vi "EGEI.vi"() -> ()   [LabVIEW 2018]
uses:
  S4GEI/S4GEI.lvclass
  S4GEI/S4GEI.lvclass/S4GEI.ctl
  Request/Request.lvclass/Request.ctl
  Command/Command.lvclass/Command.ctl
  Channel GUI/Channel.lvclass
  Command/Command.lvclass
  Camera/Camera.lvclass
  Request/Request.lvclass
panel:
  in  "Tab Control 2":enum32{"Front Panel", "Setup Panel"}(tab)
  in  "Suffix":string
  in  "Start exposure":bool
  in  "Stop Acquisition":bool
  in  "Abort Acquisition":bool
  in  "Pause acquisition":bool
  in  "Exposure time":dbl=1.5 min=9.999999747378752e-06
  in  "Frames":u16=1 min=1 max=1000
  in  "Cycles":u32=1 min=1
  in  "PROPID":string="ENG"
  in  "Observer":string="Denis"
  in  "Object name":string="Test"
  in  "comment":string
  out "Cycles done":u16(slide)=1 max=2 scale=0.0..1.0
  out "Frames done":u16(slide)=1 max=2 scale=0.0..1.0
  out "CCD Status":string
  out "Exposing":bool
  out "Last image":string
  out "Temperature":i16
  out "Serial number":u16
  out "Current exp time":dbl
  out "Used disk":i16
  out "Power":bool
  out "ACS mode":bool
  in  "Device - Fiber set":u16(ring) items=["FIBER_SET"]
  in  "Action - Fiber set":u16(ring) items=["SET"]
  in  "Parameter - Fiber set":string
  in  "Send - Fiber set":bool
  in  "Device - Camera":u16(ring) items=["RED_CHANNEL", "BLUE_CHANNEL", "BOTH_CHANNELS"]
  in  "Action - Camera":u16(ring) items=["EXPOSE", "SET_EXPTIME", "SET_FRAMES", "SET_CYCLES", "SET_SUFFIX", "ABORT_ACQUISITION", "STOP_ACQUISITION", "STOP_APP"]
  in  "Parameter - Camera":string
  in  "Send - Camera":bool
  in  "OBJECT":bool caption="object"
  in  "TEST":bool caption="test"
  in  "ZERO":bool caption="zero"
  in  "DARK":bool caption="dark"
  in  "SFLAT":bool caption="sflat"
  in  "DFLAT":bool caption="dflat"
  in  "FOCUS":bool caption="focus"
  out "Error Message":string
  in  "Stop Application":bool
  in  "Channel ID":u16=1 min=1
  in  "ACS IP":string="200.131.64.25"
  in  "Final Line":u16=2048
  in  "Final Column":u16=2048
  in  "Initial Cloumn":u16=1
  in  "Initial Line":u16=1
  in  "Binning":u16=1
  in  "Shutter TTL":u16(ring) items=["TTL Low", "TTL High", "Error"]
  in  "Shutter Time":u16=50
  in  "Shutter Mode":u8(ring)=2 items=["OPEN"=1, "CLOSED"=2, "Error"=3]
  in  "AD Channel":u16
  in  "VShift Speed":u16(ring) items=["38.55", "76.95", "Error"]
  in  "Trigger Mode":u16(ring) items=["Internal", "External", "N/A", "N/A", "N/A", "N/A", "External Start", "External Exposure (Bulb)", "N/A", "External FVB EM", "Software", "N/A", "External Charge Shifting"]
  in  "Read Mode":u16(ring)=4 items=["Full Vertical Binning", "Multi-Track", "Random-Track", "Single-Track", "Image"]
  in  "Clock Amplitude":u16(ring) items=["Normal", "+1", "+2", "+3", "+4", "Error"]
  in  "Set camera configuration":bool
  in  "Temp":i32=20 min=-80 max=20
  in  "Cooler":bool
  in  "Sub Image":T1(radio)=enum."2048 x 2048"
  in  "High capacity":u16(ring) items=["Disabled", "Enabled"]
  in  "Readout Rate":u8(ring) items=["50 KHz", "1 MHz", "3 MHz", "5 MHz"]
  in  "Pre-amp gain":u8(ring) items=["Gain 1", "Gain 2", "Gain 4", "Error"]
  in  "Acquisition Mode":u16(ring)=3 items=["Reserved", "Single Scan", "Accumulate", "Kinetic", "Fast Kinetic", "Run till abort", "Reserved", "Reserved", "Reserved", "Time Delayed Integration"]
  # "ECHARPE Graphical Engineering Interface (EGEI)"
  # "Observation info"
  # "Request"
  # "Acquisition control"
  # "Pre-sets"
  # "Camera status"
  # "Errors"
  # "Camera operation mode"
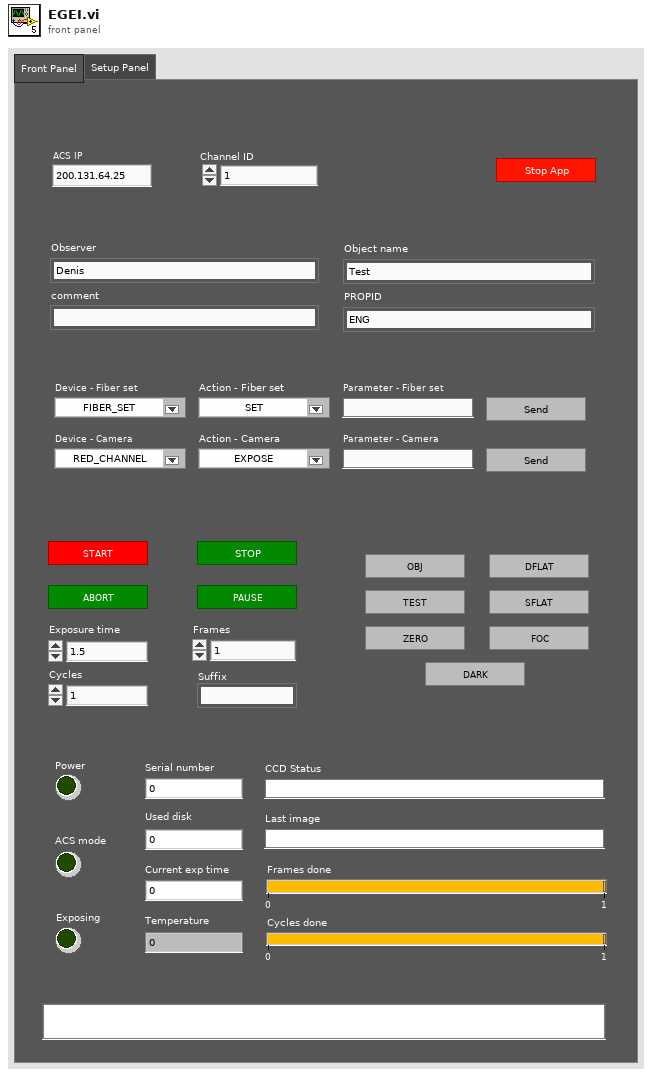
[diagram p1: front panel]
types:
  T1 = enum32{"512 x 512", "1024 x 1024", "Custom", "2048 x 2048"}
  T2 = cluster{"FWCS IP":string, "ACS IP":string, "Channel ID":u16}
  T3 = enum8{"Enabled", "Disabled", "Disabled and Grayed Out"}
  T4 = cluster{"CYCLES_DONE":u16, "LAST_IMAGE_NAME":string, "USED_DISK_SPACE":u16, "FRAMES_DONE":u16, "CCD_STATUS":string, "CURRENT_TEMPERATURE":i16, "TEMPERATURE_STATUS":string, "FRAME_EXPOSURE_TIME":sgl, "SERIAL_NUMBER":u16, "ACQUIRING":bool, "IMAGE_INDEX":u32, "POWER":bool, "ACS MODE":bool}
  T5 = cluster{"State Machine.lvclass":refnum<class "State Machine.lvclass">, "Channel.lvclass":refnum<class "Channel.lvclass">, "STATUS.lvclass":refnum<class "RxTx.lvclass">, "Status SM.lvclass":refnum<class "State Machine.lvclass">, "S4ICS.lvclass":refnum<class "S4ICS.lvclass">, "Acq State Machine.lvclass":refnum<class "State Machine.lvclass">, "Request SM.lvclass":refnum<class "State Machine.lvclass">, "Request.lvclass":refnum<class "Request.lvclass">}
  T6 = cluster{"device":string, "action":string, "parameter":string}
  T7 = cluster{"PREAMP":u16, "READOUT_RATE":u16, "VERTICAL_SHIFT_SPEED":u16, "READ_MODE":u16, "VERTICAL_CLOCK_VOLTAGE":u16, "ACQUISITION_MODE":u16, "AD_CHANNEL":u16, "SHUTTER_TTL":u16, "SHUTTER_OPENING_TIME":u16, "SHUTTER_CLOSING_TIME":u16, "SHUTTER_MODE":u16, "TRIGGER_MODE":u16, "VBIN":u16, "INITIAL_LINE":u16, "INITIAL_COLUMN":u16, "FINAL_LINE":u16, "FINAL_COLUMN":u16, "HBIN":u16, "HIGH_CAPACITY":bool, "COOLER":u16, "TEMP":u16}
  T8 = cluster{"EXPTIME":dbl, "#FRAMES":u32, "#CYCLES":u32, "suffix":string}
  T9 = cluster{"OBJECT":string, "OBSERVER":string, "CTRLINTE":string, "PROJID":string, "SYNCMODE":string, "INSTMODE":string, "FILTER":string, "OBSTYPE":string, "GUIVRSN":string, "COMMENT":string, "broker":string, "timestamp":string, "CHANNEL 1":bool, "CHANNEL 2":bool, "CHANNEL 3":bool, "CHANNEL 4":bool, "TCSMODE":bool}
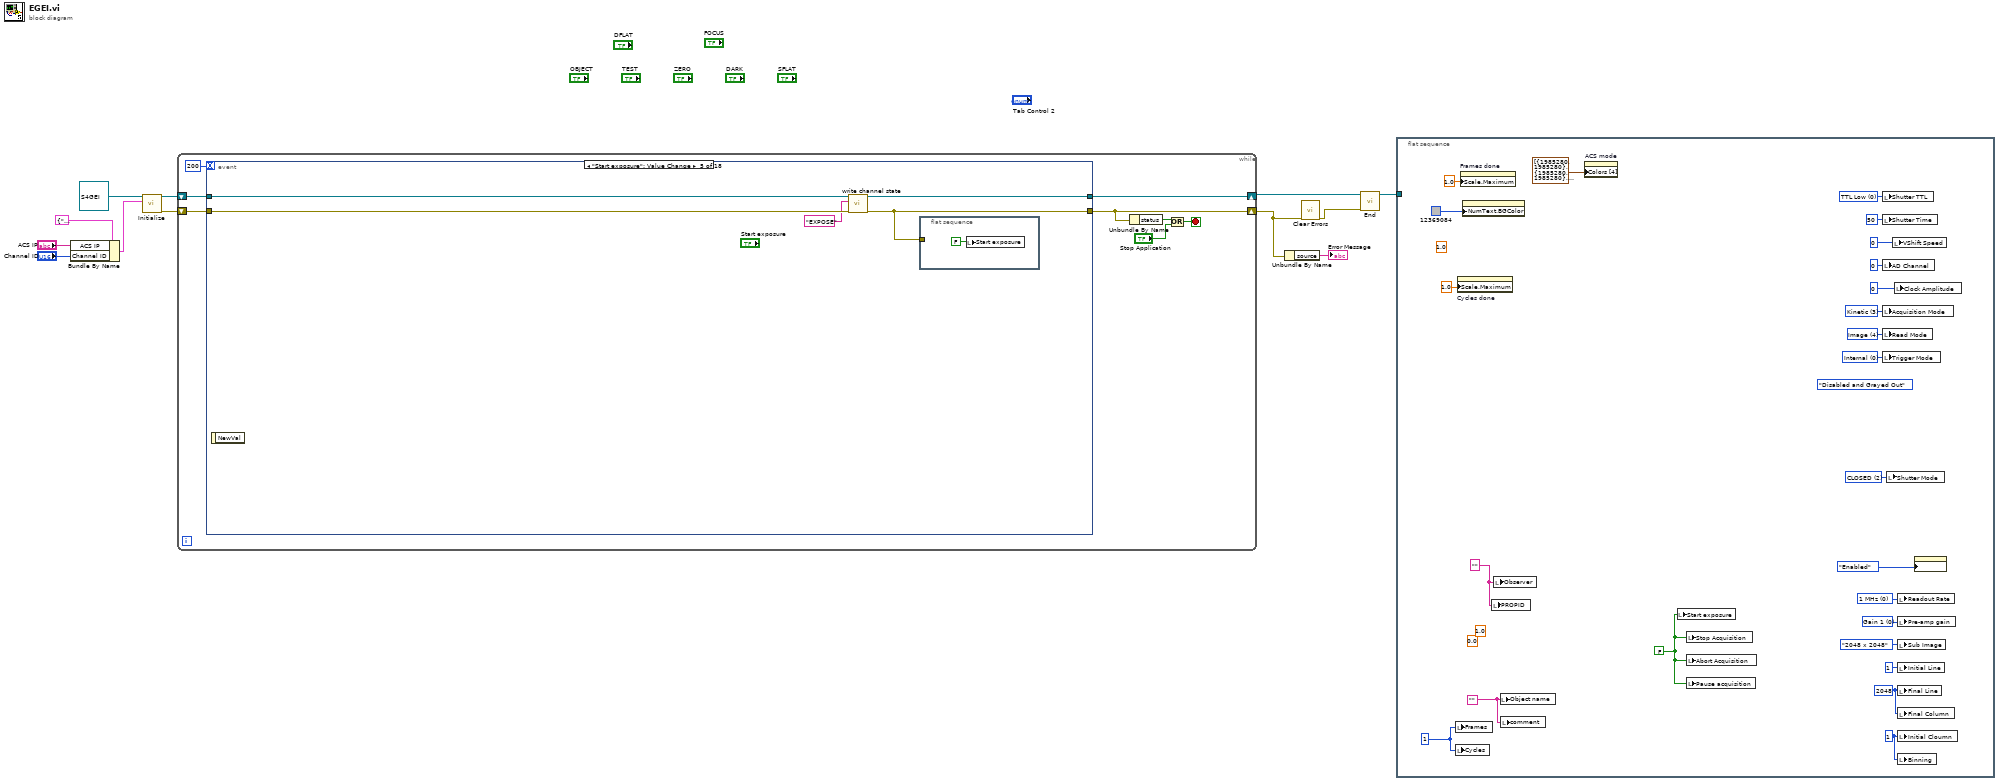
[diagram p0: block diagram]
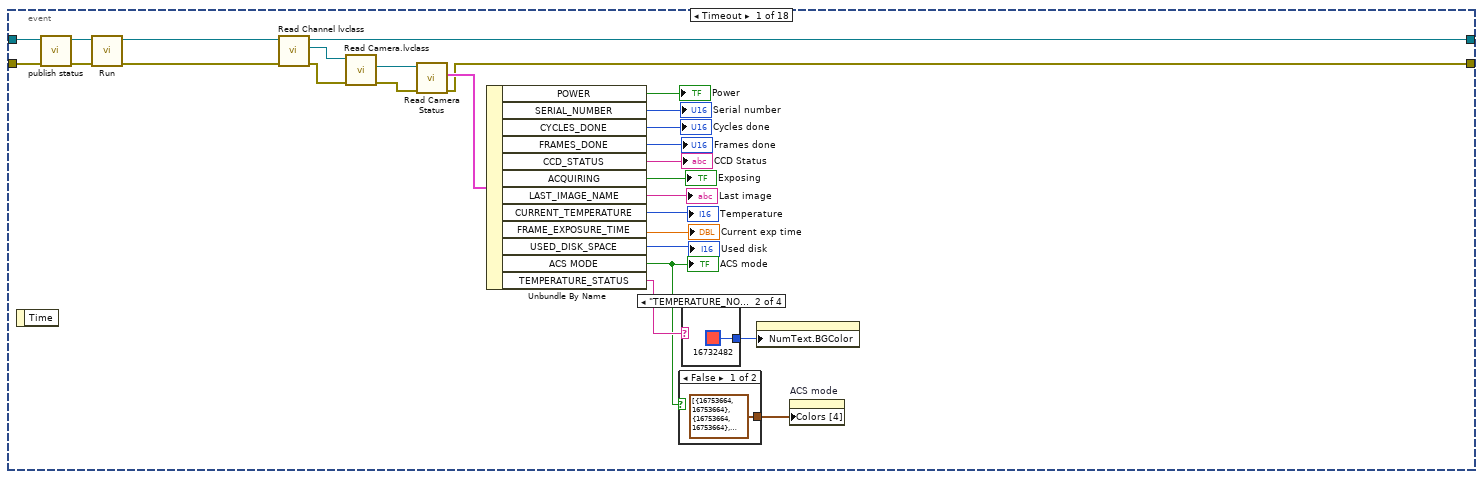
[diagram p2: hidden frame]
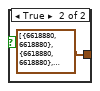
[diagram p3: hidden frame]
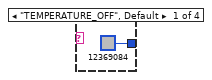
[diagram p4: hidden frame]
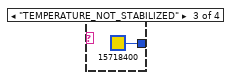
[diagram p5: hidden frame]
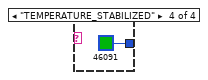
[diagram p6: hidden frame]
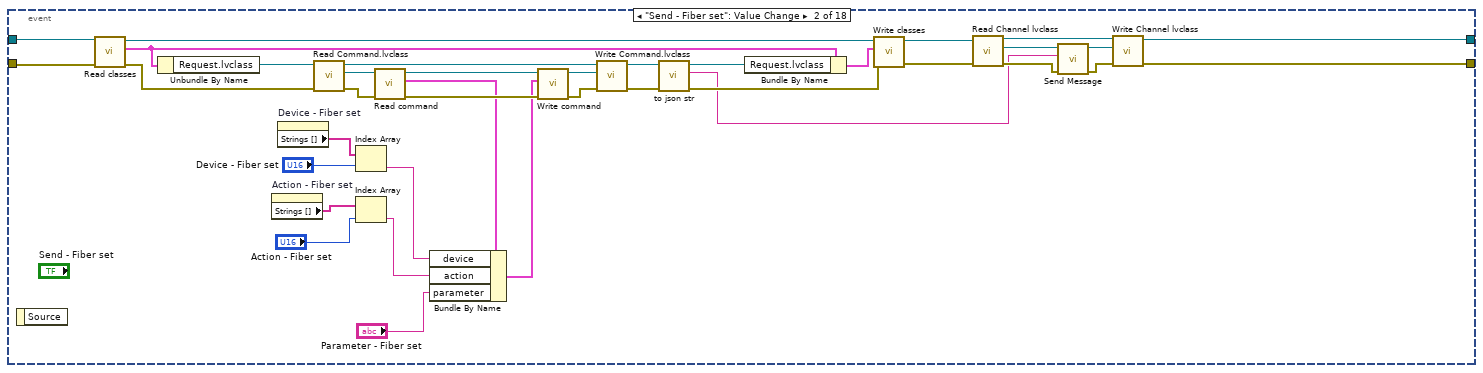
[diagram p7: hidden frame]
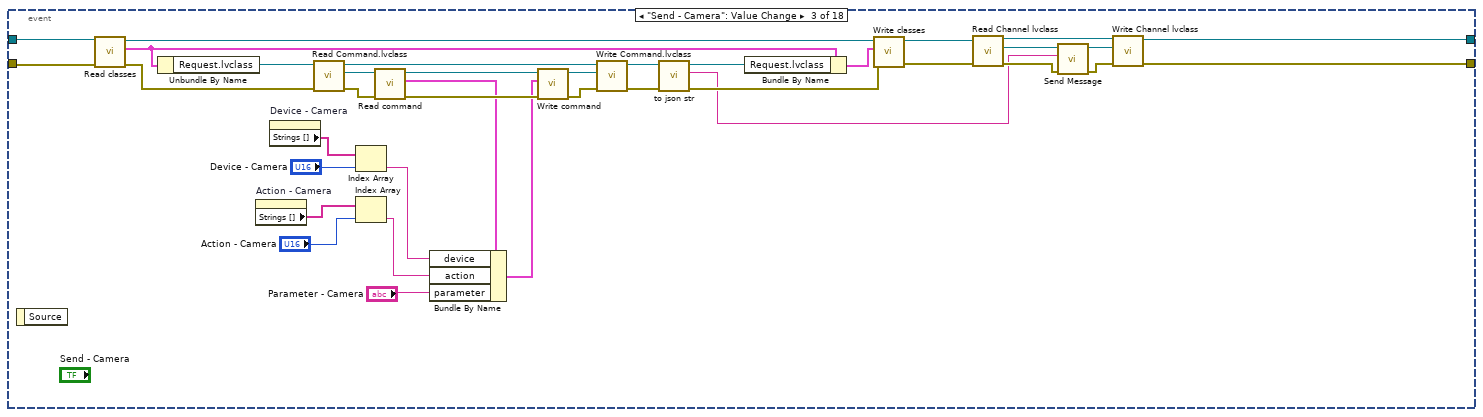
[diagram p8: hidden frame]
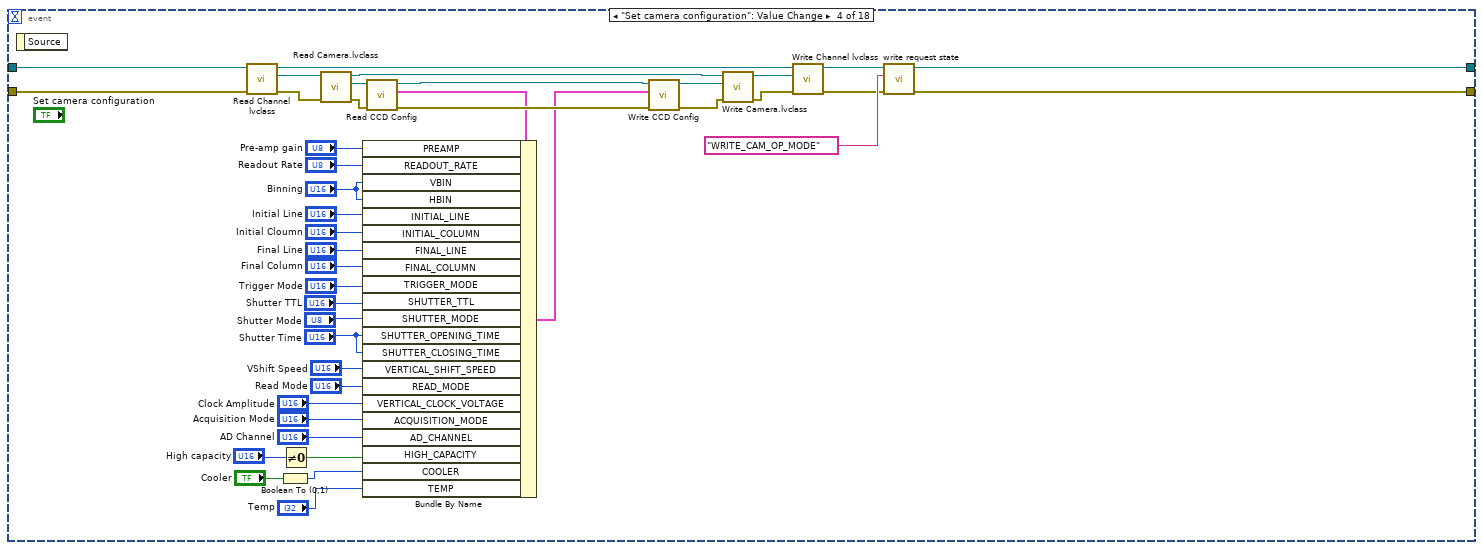
[diagram p9: hidden frame]
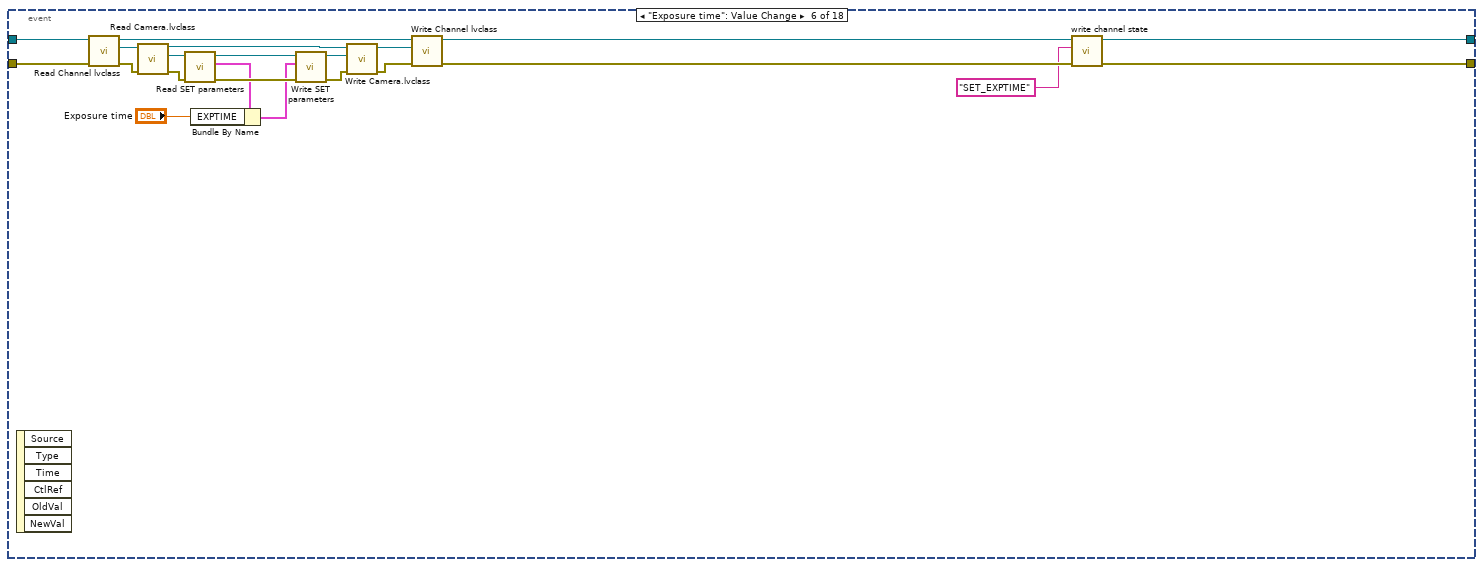
[diagram p10: hidden frame]
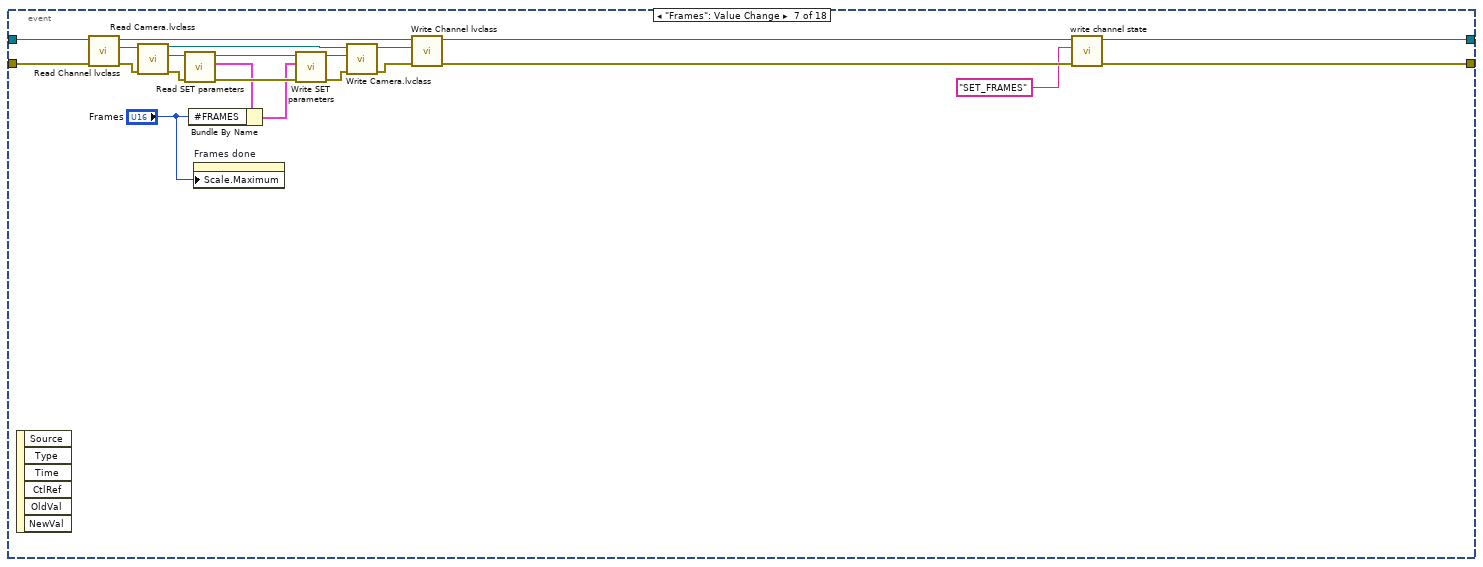
[diagram p11: hidden frame]
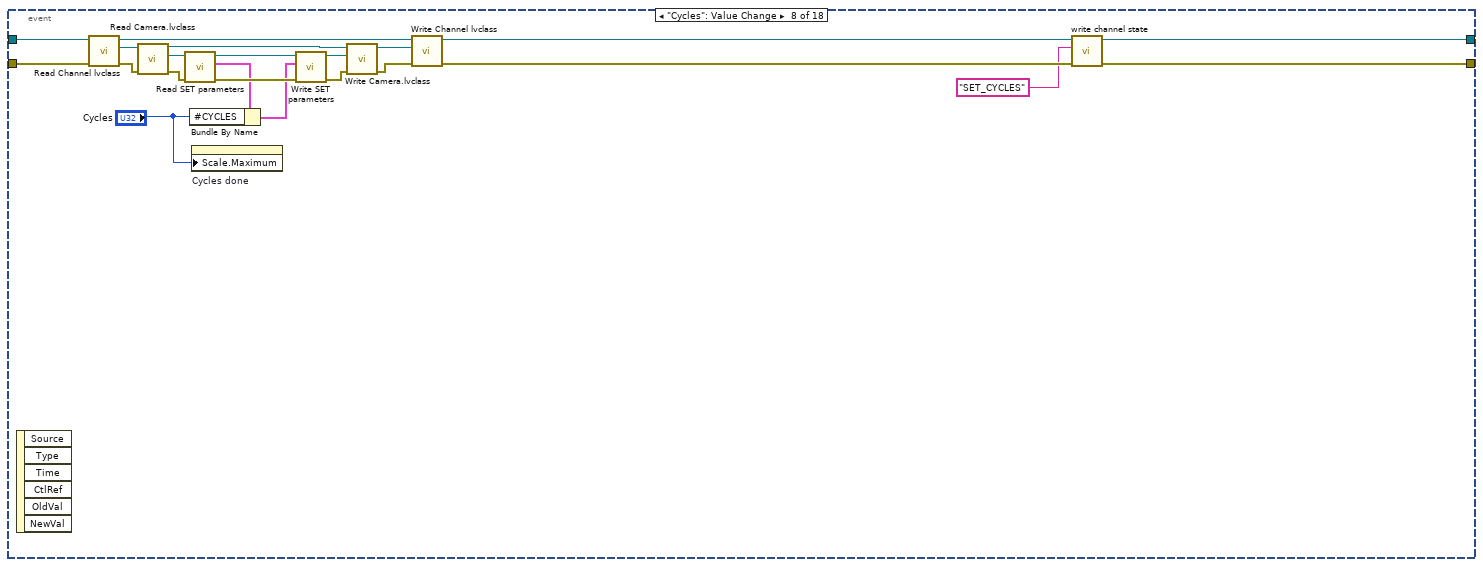
[diagram p12: hidden frame]
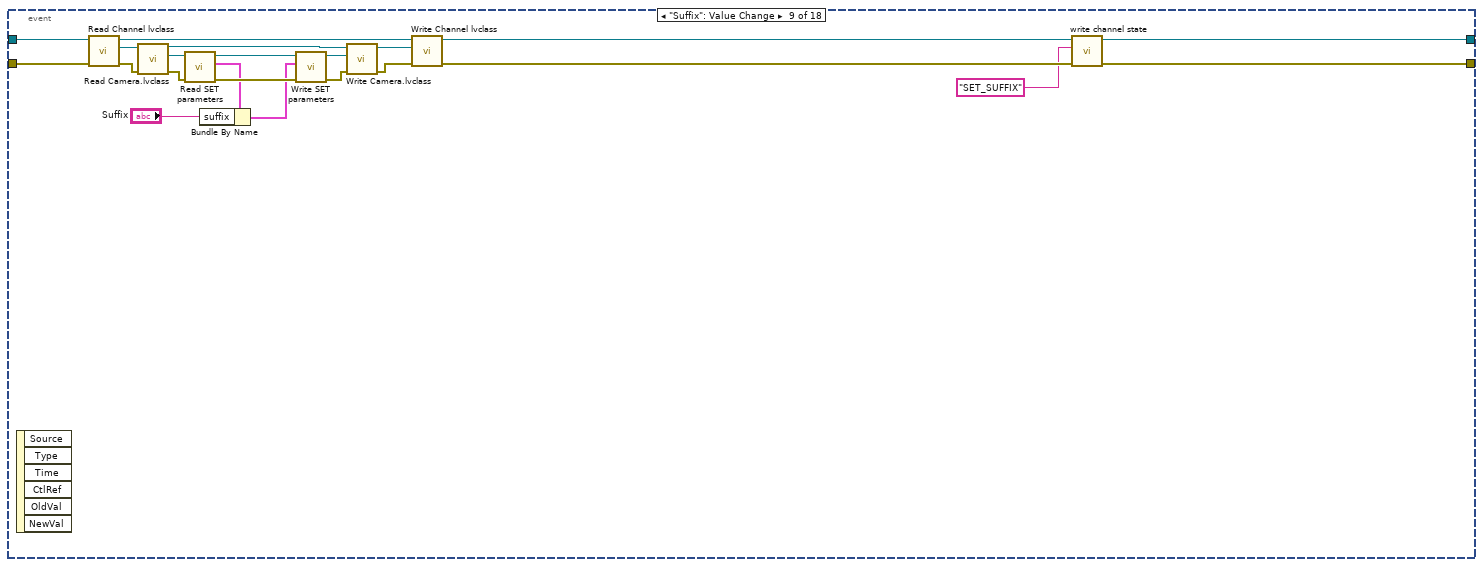
[diagram p13: hidden frame]
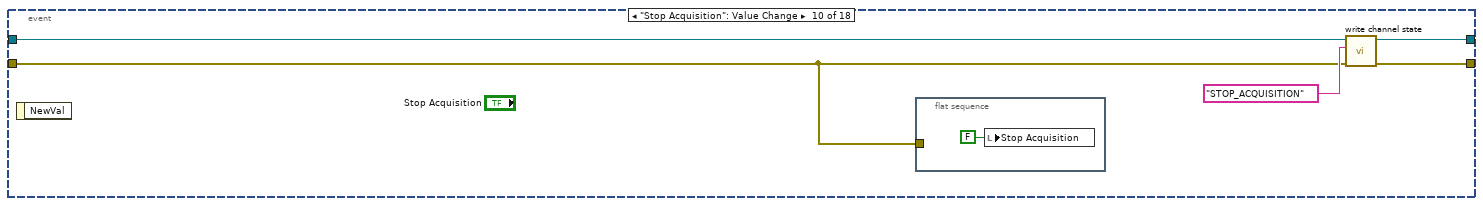
[diagram p14: hidden frame]
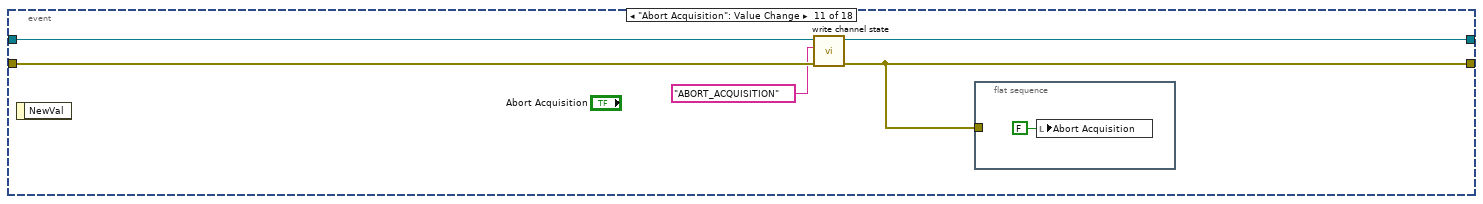
[diagram p15: hidden frame]
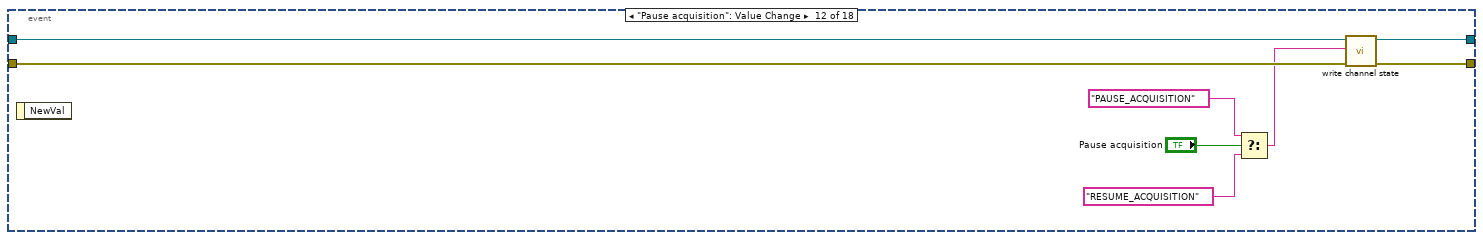
[diagram p16: hidden frame]
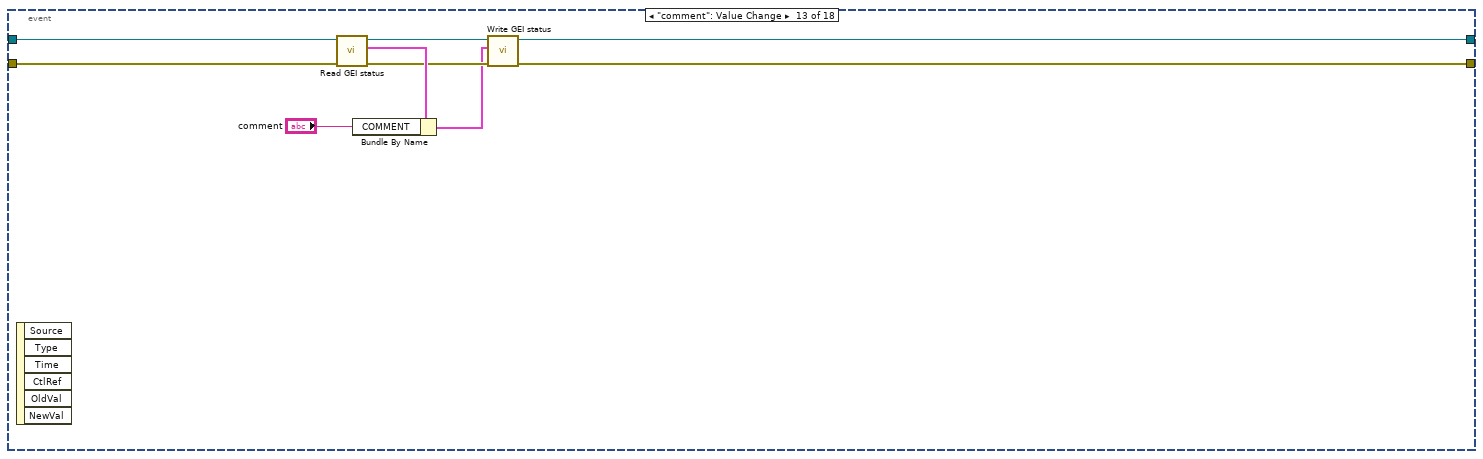
[diagram p17: hidden frame]
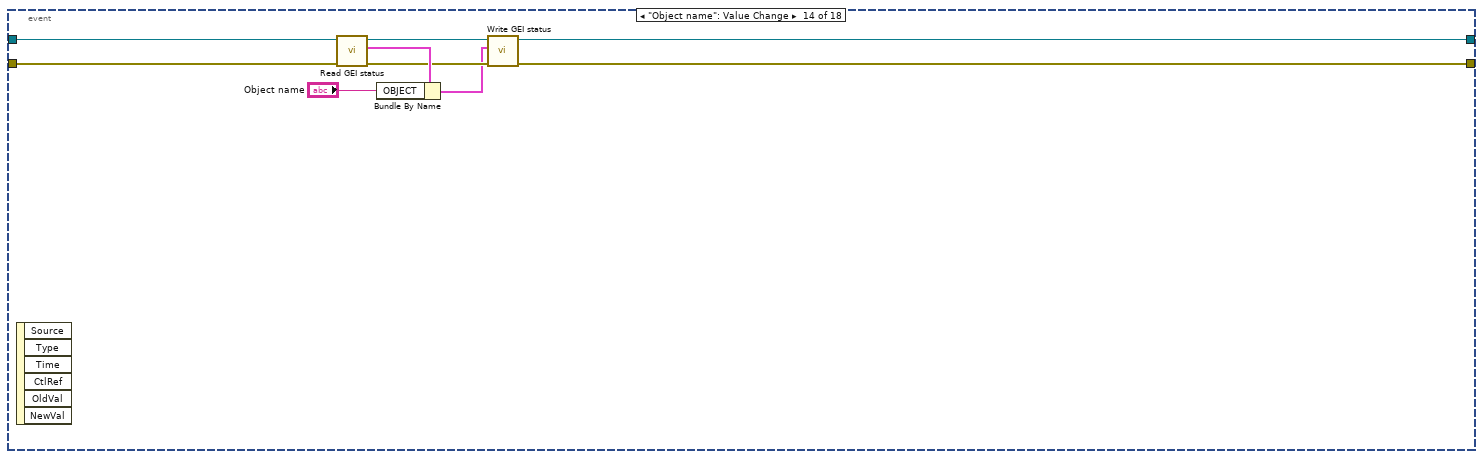
[diagram p18: hidden frame]
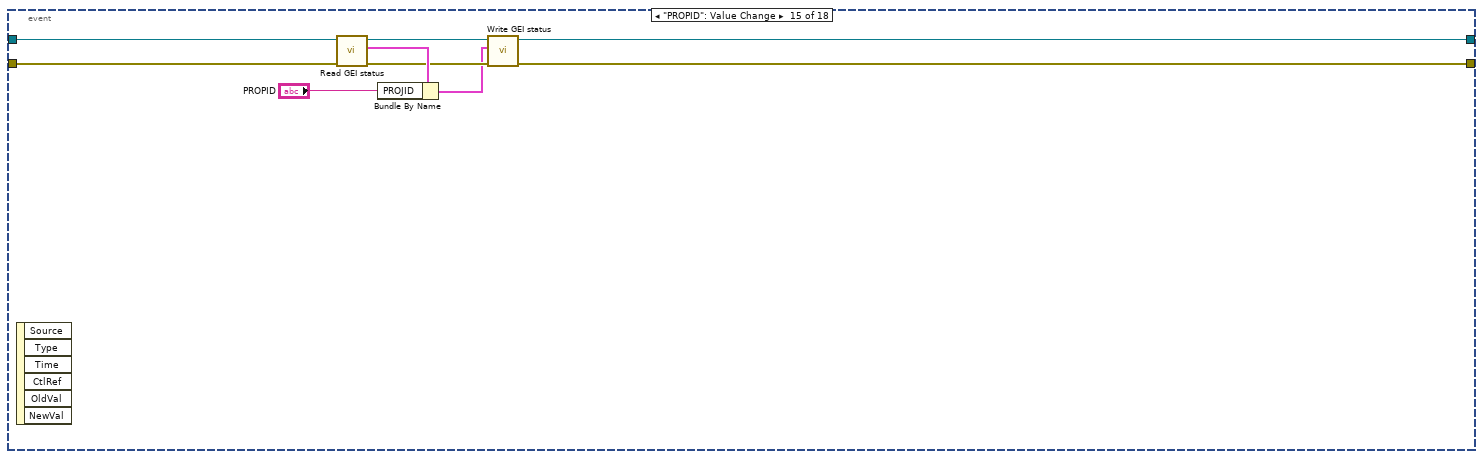
[diagram p19: hidden frame]
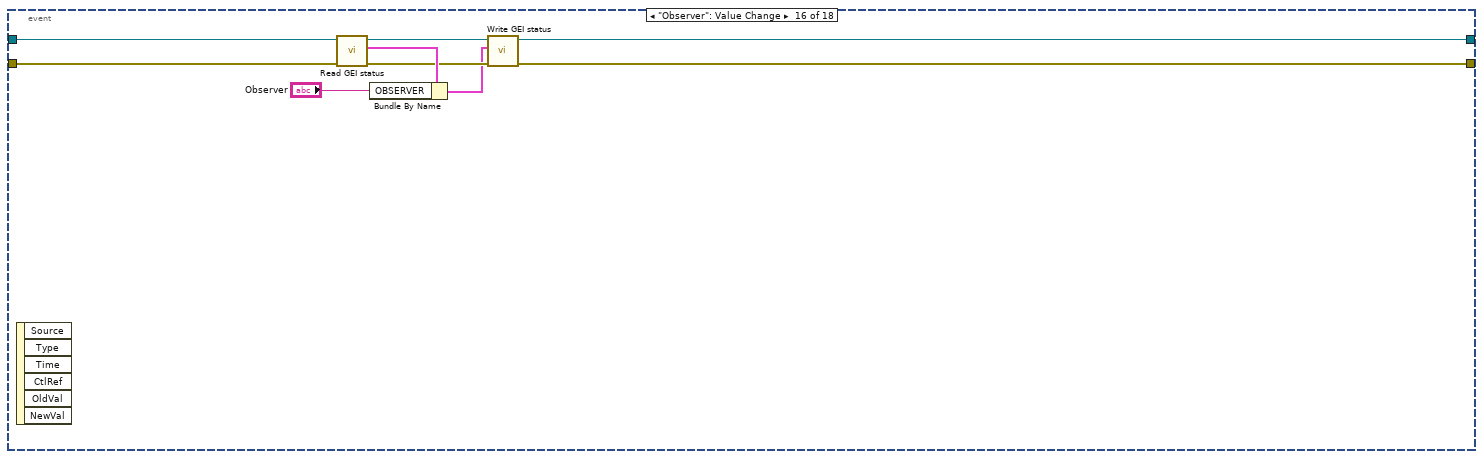
[diagram p20: hidden frame]
diagram:
  n1 = Bundle By Name(cluster=T2 {"FWCS IP"="200.131.64.49", "ACS IP"="200.131.64.25", "Channel ID"=1} ("Communication variables"), "ACS IP"="ACS IP", "Channel ID"="Channel ID") -> (w6:T2)
  n2 = call "Initialize.vi"("Communication variables"=w6, "SPARC4_GUI in"=refnum<class "S4GEI.lvclass"> refnum ("SPARC4_GUI.lvclass")) -> ("error out"=w2:errorcluster, "SPARC4_GUI out"=w1:refnum<class "S4GEI.lvclass">)  [unwired: 8 in]
  n3 = while {
    shift-right: [w13] -> w9
    shift-left: w2 -> [w15]
    shift-right: [w14] -> w11
    shift-left: w1 -> [w16]
    stop <- w19 stop-if-true
    n4 = event shown="[4] \"Start exposure\": Value Change" {
      selector: _ -> [_ _ _ _ _ _ _ _ _ _ _ _ _ _ _ _ _ _]
      dyn-events: _ -> [_ _ _ _ _ _ _ _ _ _ _ _ _ _ _ _ _ _]
      timeout: 200 -> [_ _ _ _ _ _ _ _ _ _ _ _ _ _ _ _ _ _]
      tunnel: w15 -> [w44 w70 w107 w168 w173 w195 w217 w239 w261 w264 w273 w282 w289 w298 w307 w316 w334 w357]
      tunnel: [w36 w84 w121 w134 w170 w177 w199 w221 w243 w266 w270 w280 w290 w299 w308 w317 w332 w357] -> w13
      tunnel: w16 -> [w45 w71 w108 w169 w174 w196 w218 w240 w262 w268 w274 w283 w291 w300 w309 w318 w335 w356]
      tunnel: [w37 w85 w122 w133 w171 w178 w200 w222 w244 w267 w272 w281 w292 w301 w310 w319 w333 w356] -> w14
      event Timeout {
        n5 = event-data() -> ()  [unwired: 1 in, 1 out]
        n6 = call "publish status.vi"("error in (no error)"=w44, "S4GEI in"=w45) -> ("error out"=w43:errorcluster, "S4GEI out"=w42:refnum<class "S4GEI.lvclass">)  [unwired: 8 in]
        n7 = call "Run.vi"("error in (no error)"=w43, "SPARC4_GUI in"=w42) -> ("error out"=w34:errorcluster, "SPARC4_GUI out"=w35:refnum<class "S4GEI.lvclass">)  [unwired: 8 in]
        n8 = call "Read Channel lvclass.vi"("error in (no error)"=w34, "SPARC4_GUI in"=w35) -> ("error out"=w39:errorcluster, "Channel.lvclass"=w41:refnum<class "Channel.lvclass">, "SPARC4_GUI out"=w37:refnum<class "S4GEI.lvclass">)  [unwired: 7 in]
        n9 = call-dynamic "Read Camera.lvclass.vi"("error in (no error)"=w39, "Channel in"=w41) -> ("error out"=w38:errorcluster, "Camera.lvclass"=w40:refnum<class "Camera.lvclass">)  [unwired: 7 in, 1 out]
        n10 = call-dynamic "Read Camera Status.vi"("error in (no error)"=w38, "Camera in"=w40) -> ("error out"=w36:errorcluster, "camera status"=w46:T4)  [unwired: 7 in, 1 out]
        n11 = Unbundle By Name(w46) -> ("POWER"=→"Power":bool, "SERIAL_NUMBER"=→"Serial number":u16, "CYCLES_DONE"=→"Cycles done":u16, "FRAMES_DONE"=→"Frames done":u16, "CCD_STATUS"=→"CCD Status":string, "ACQUIRING"=→"Exposing":bool, "LAST_IMAGE_NAME"=→"Last image":string, "CURRENT_TEMPERATURE"=→"Temperature":i16, "FRAME_EXPOSURE_TIME"=→"Current exp time":sgl, "USED_DISK_SPACE"=→"Used disk":u16, "ACS MODE"=w29:bool, "TEMPERATURE_STATUS"=w33:string)
        "ACS mode" <- w29
        n12 = case shown="False" w29 {
          tunnel: [cluster{u32, u32}[] [{16753664, 16753664}, {16753664, 16753664}, {16753664, 16753664}] ("Colors [4]") cluster{u32, u32}[] [{6618880, 6618880}, {6618880, 6618880}, {6618880, 6618880}] ("Colors [4]")] -> w32
          frame False {
          }
          frame True {
          }
        }
        n13 = case shown="\"TEMPERATURE_NOT_REACHED\"" w33 {
          tunnel: [u32 12369084 u32 16732482 u32 15718400 u32 46091] -> w47
          frame "TEMPERATURE_OFF", Default {
          }
          frame "TEMPERATURE_NOT_REACHED" {
          }
          frame "TEMPERATURE_NOT_STABILIZED" {
          }
          frame "TEMPERATURE_STABILIZED" {
          }
        }
        n14 = property on="Temperature" class="DigNum (strict)"("NumText.BGColor"=w47) -> ()  [unwired: 2 in, 2 out]
        n15 = property on="ACS mode" class="Bool (strict)"("Colors [4]"=w32) -> ()  [unwired: 2 in, 2 out]
      }
      event "Send - Fiber set": Value Change {
        n16 = event-data() -> ()  [unwired: 1 in, 1 out]
        n17 = call-dynamic "Read classes.vi"("error in (no error)"=w70, "S4GEI in"=w71) -> ("error out"=w72:errorcluster, "classes"=w81:T5, "S4GEI out"=w79:refnum<class "S4GEI.lvclass">)  [unwired: 7 in]
        n18 = Unbundle By Name(w81) -> ("Request.lvclass"=w83:refnum<class "Request.lvclass">)
        n19 = property on="Action - Fiber set" class="Ring (strict)"() -> ("Strings []"=w56:string[])  [unwired: 2 in, 2 out]
        n20 = property on="Device - Fiber set" class="Ring (strict)"() -> ("Strings []"=w59:string[])  [unwired: 2 in, 2 out]
        n21 = call "Read Command.lvclass.vi"("error in (no error)"=w72, "Request in"=w83) -> ("error out"=w73:errorcluster, "Command.lvclass"=w78:refnum<class "Command.lvclass">, "Request out"=w82:refnum<class "Request.lvclass">)  [unwired: 7 in]
        n22 = Index Array(array=w59, index="Device - Fiber set") -> (element=w58:string)
        n23 = Index Array(array=w56, index="Action - Fiber set") -> (element=w54:string)
        n24 = call "Read command.vi"("error in (no error)"=w73, "Command in"=w78) -> ("error out"=w74:errorcluster, "command"=w67:T6, "Command out"=w77:refnum<class "Command.lvclass">)  [unwired: 7 in]
        n25 = Bundle By Name(cluster=w67, "device"=w58, "action"=w54, "parameter"="Parameter - Fiber set") -> (w66:T6)
        n26 = call "Write command.vi"("error in (no error)"=w74, "command"=w66, "Command in"=w77) -> ("error out"=w75:errorcluster, "Command out"=w76:refnum<class "Command.lvclass">)  [unwired: 7 in]
        n27 = call "Write Command.lvclass.vi"("error in (no error)"=w75, "Command.lvclass"=w76, "Request in"=w82) -> ("error out"=w63:errorcluster, "Request out"=w64:refnum<class "Request.lvclass">)  [unwired: 7 in]
        n28 = call "to json str.vi"("error in (no error)"=w63, "Request in"=w64) -> ("error out"=w62:errorcluster, "request str"=w60:string, "Request out"=w61:refnum<class "Request.lvclass">)  [unwired: 7 in]
        n29 = Bundle By Name(cluster=w81, "Request.lvclass"=w61) -> (w80:T5)
        n30 = call-dynamic "Write classes.vi"("error in (no error)"=w62, "classes"=w80, "S4GEI in"=w79) -> ("error out"=w68:errorcluster, "S4GEI out"=w69:refnum<class "S4GEI.lvclass">)  [unwired: 7 in]
        n31 = call "Read Channel lvclass.vi"("error in (no error)"=w68, "SPARC4_GUI in"=w69) -> ("error out"=w87:errorcluster, "Channel.lvclass"=w90:refnum<class "Channel.lvclass">, "SPARC4_GUI out"=w86:refnum<class "S4GEI.lvclass">)  [unwired: 7 in]
        n32 = call "Send Message.vi"("error in (no error)"=w87, "Message"=w60, "Channel GUI in"=w90) -> ("error out"=w88:errorcluster, "Channel GUI out"=w89:refnum<class "Channel.lvclass">)  [unwired: 7 in]
        n33 = call "Write Channel lvclass.vi"("error in (no error)"=w88, "Channel.lvclass"=w89, "SPARC4_GUI in"=w86) -> ("error out"=w84:errorcluster, "SPARC4_GUI out"=w85:refnum<class "S4GEI.lvclass">)  [unwired: 7 in]
      }
      event "Send - Camera": Value Change {
        n34 = event-data() -> ()  [unwired: 1 in, 1 out]
        n35 = call-dynamic "Read classes.vi"("error in (no error)"=w107, "S4GEI in"=w108) -> ("error out"=w109:errorcluster, "classes"=w118:T5, "S4GEI out"=w116:refnum<class "S4GEI.lvclass">)  [unwired: 7 in]
        n36 = Unbundle By Name(w118) -> ("Request.lvclass"=w120:refnum<class "Request.lvclass">)
        n37 = property on="Action - Camera" class="Ring (strict)"() -> ("Strings []"=w93:string[])  [unwired: 2 in, 2 out]
        n38 = property on="Device - Camera" class="Ring (strict)"() -> ("Strings []"=w95:string[])  [unwired: 2 in, 2 out]
        n39 = call "Read Command.lvclass.vi"("error in (no error)"=w109, "Request in"=w120) -> ("error out"=w110:errorcluster, "Command.lvclass"=w115:refnum<class "Command.lvclass">, "Request out"=w119:refnum<class "Request.lvclass">)  [unwired: 7 in]
        n40 = Index Array(array=w95, index="Device - Camera") -> (element=w91:string)
        n41 = Index Array(array=w93, index="Action - Camera") -> (element=w92:string)
        n42 = call "Read command.vi"("error in (no error)"=w110, "Command in"=w115) -> ("error out"=w111:errorcluster, "command"=w104:T6, "Command out"=w114:refnum<class "Command.lvclass">)  [unwired: 7 in]
        n43 = Bundle By Name(cluster=w104, "device"=w91, "action"=w92, "parameter"="Parameter - Camera") -> (w103:T6)
        n44 = call "Write command.vi"("error in (no error)"=w111, "command"=w103, "Command in"=w114) -> ("error out"=w112:errorcluster, "Command out"=w113:refnum<class "Command.lvclass">)  [unwired: 7 in]
        n45 = call "Write Command.lvclass.vi"("error in (no error)"=w112, "Command.lvclass"=w113, "Request in"=w119) -> ("error out"=w101:errorcluster, "Request out"=w102:refnum<class "Request.lvclass">)  [unwired: 7 in]
        n46 = call "to json str.vi"("error in (no error)"=w101, "Request in"=w102) -> ("error out"=w100:errorcluster, "request str"=w98:string, "Request out"=w99:refnum<class "Request.lvclass">)  [unwired: 7 in]
        n47 = Bundle By Name(cluster=w118, "Request.lvclass"=w99) -> (w117:T5)
        n48 = call-dynamic "Write classes.vi"("error in (no error)"=w100, "classes"=w117, "S4GEI in"=w116) -> ("error out"=w105:errorcluster, "S4GEI out"=w106:refnum<class "S4GEI.lvclass">)  [unwired: 7 in]
        n49 = call "Read Channel lvclass.vi"("error in (no error)"=w105, "SPARC4_GUI in"=w106) -> ("error out"=w124:errorcluster, "Channel.lvclass"=w127:refnum<class "Channel.lvclass">, "SPARC4_GUI out"=w123:refnum<class "S4GEI.lvclass">)  [unwired: 7 in]
        n50 = call "Send Message.vi"("error in (no error)"=w124, "Message"=w98, "Channel GUI in"=w127) -> ("error out"=w125:errorcluster, "Channel GUI out"=w126:refnum<class "Channel.lvclass">)  [unwired: 7 in]
        n51 = call "Write Channel lvclass.vi"("error in (no error)"=w125, "Channel.lvclass"=w126, "SPARC4_GUI in"=w123) -> ("error out"=w121:errorcluster, "SPARC4_GUI out"=w122:refnum<class "S4GEI.lvclass">)  [unwired: 7 in]
      }
      event "Set camera configuration": Value Change {
        n52 = event-data() -> ()  [unwired: 1 in, 1 out]
        n53 = call "Read Channel lvclass.vi"("error in (no error)"=w168, "SPARC4_GUI in"=w169) -> ("error out"=w167:errorcluster, "Channel.lvclass"=w139:refnum<class "Channel.lvclass">, "SPARC4_GUI out"=w166:refnum<class "S4GEI.lvclass">)  [unwired: 7 in]
        n54 = Boolean To (0,1)(Boolean="Cooler") -> (0, 1=w131:i16)
        n55 = Not Equal To 0?(x="High capacity") -> (x != 0?=w128:bool)
        n56 = call-dynamic "Read Camera.lvclass.vi"("error in (no error)"=w167, "Channel in"=w139) -> ("error out"=w165:errorcluster, "Camera.lvclass"=w164:refnum<class "Camera.lvclass">, "Channel out"=w138:refnum<class "Channel.lvclass">)  [unwired: 7 in]
        n57 = call-dynamic "Read CCD Config.vi"("error in (no error)"=w165, "Camera in"=w164) -> ("error out"=w163:errorcluster, "CCD Config"=w141:T7, "Camera out"=w146:refnum<class "Camera.lvclass">)  [unwired: 7 in]
        n58 = Bundle By Name(cluster=w141, "PREAMP"="Pre-amp gain", "READOUT_RATE"="Readout Rate", "VBIN"="Binning", "HBIN"="Binning", "INITIAL_LINE"="Initial Line", "INITIAL_COLUMN"="Initial Cloumn", "FINAL_LINE"="Final Line", "FINAL_COLUMN"="Final Column", "TRIGGER_MODE"="Trigger Mode", "SHUTTER_TTL"="Shutter TTL", "SHUTTER_MODE"="Shutter Mode", "SHUTTER_OPENING_TIME"="Shutter Time", "SHUTTER_CLOSING_TIME"="Shutter Time", "VERTICAL_SHIFT_SPEED"="VShift Speed", "READ_MODE"="Read Mode", "VERTICAL_CLOCK_VOLTAGE"="Clock Amplitude", "ACQUISITION_MODE"="Acquisition Mode", "AD_CHANNEL"="AD Channel", "HIGH_CAPACITY"=w128, "COOLER"=w131, "TEMP"="Temp") -> (w140:T7)
        n59 = call-dynamic "Write CCD Config.vi"("error in (no error)"=w163, "CCD Config"=w140, "Camera in"=w146) -> ("error out"=w144:errorcluster, "Camera out"=w145:refnum<class "Camera.lvclass">)  [unwired: 7 in]
        n60 = call-dynamic "Write Camera.lvclass.vi"("error in (no error)"=w144, "Camera.lvclass"=w145, "Channel in"=w138) -> ("error out"=w143:errorcluster, "Channel out"=w142:refnum<class "Channel.lvclass">)  [unwired: 7 in]
        n61 = call "Write Channel lvclass.vi"("error in (no error)"=w143, "Channel.lvclass"=w142, "SPARC4_GUI in"=w166) -> ("error out"=w136:errorcluster, "SPARC4_GUI out"=w135:refnum<class "S4GEI.lvclass">)  [unwired: 7 in]
        n62 = call "write request state.vi"("error in (no error)"=w136, "State"="WRITE_CAM_OP_MODE", "S4GEI in"=w135) -> ("error out"=w134:errorcluster, "S4GEI out"=w133:refnum<class "S4GEI.lvclass">)  [unwired: 7 in]
      }
      event "Start exposure": Value Change {
        n63 = event-data() -> ()  [unwired: 1 in, 1 out]
        n64 = call "write channel state.vi"("error in (no error)"=w173, "State"="EXPOSE", "S4GEI in"=w174) -> ("error out"=w170:errorcluster, "S4GEI out"=w171:refnum<class "S4GEI.lvclass">)  [unwired: 7 in]
        n65 = flat-sequence {
          tunnel: w170 -> [_]
          frame #0 {
            n66 = local write "Start exposure"(FALSE ("Start exposure")) -> ()
          }
        }
      }
      event "Exposure time": Value Change {
        n67 = event-data() -> ()  [unwired: 1 in, 6 out]
        n68 = call "Read Channel lvclass.vi"("error in (no error)"=w195, "SPARC4_GUI in"=w196) -> ("error out"=w194:errorcluster, "Channel.lvclass"=w183:refnum<class "Channel.lvclass">, "SPARC4_GUI out"=w197:refnum<class "S4GEI.lvclass">)  [unwired: 7 in]
        n69 = call-dynamic "Read Camera.lvclass.vi"("error in (no error)"=w194, "Channel in"=w183) -> ("error out"=w190:errorcluster, "Camera.lvclass"=w191:refnum<class "Camera.lvclass">, "Channel out"=w182:refnum<class "Channel.lvclass">)  [unwired: 7 in]
        n70 = call-dynamic "Read SET parameters.vi"("error in (no error)"=w190, "Camera in"=w191) -> ("error out"=w188:errorcluster, "SET parameters"=w185:T8, "Camera out"=w189:refnum<class "Camera.lvclass">)  [unwired: 7 in]
        n71 = Bundle By Name(cluster=w185, "EXPTIME"="Exposure time") -> (w184:T8)
        n72 = call-dynamic "Write SET parameters.vi"("error in (no error)"=w188, "SET parameters"=w184, "Camera in"=w189) -> ("error out"=w186:errorcluster, "Camera out"=w187:refnum<class "Camera.lvclass">)  [unwired: 7 in]
        n73 = call-dynamic "Write Camera.lvclass.vi"("error in (no error)"=w186, "Camera.lvclass"=w187, "Channel in"=w182) -> ("error out"=w193:errorcluster, "Channel out"=w192:refnum<class "Channel.lvclass">)  [unwired: 7 in]
        n74 = call "Write Channel lvclass.vi"("error in (no error)"=w193, "Channel.lvclass"=w192, "SPARC4_GUI in"=w197) -> ("error out"=w180:errorcluster, "SPARC4_GUI out"=w181:refnum<class "S4GEI.lvclass">)  [unwired: 7 in]
        n75 = call "write channel state.vi"("error in (no error)"=w180, "State"="SET_EXPTIME", "S4GEI in"=w181) -> ("error out"=w177:errorcluster, "S4GEI out"=w178:refnum<class "S4GEI.lvclass">)  [unwired: 7 in]
      }
      event "Frames": Value Change {
        n76 = event-data() -> ()  [unwired: 1 in, 6 out]
        n77 = call "Read Channel lvclass.vi"("error in (no error)"=w217, "SPARC4_GUI in"=w218) -> ("error out"=w216:errorcluster, "Channel.lvclass"=w205:refnum<class "Channel.lvclass">, "SPARC4_GUI out"=w219:refnum<class "S4GEI.lvclass">)  [unwired: 7 in]
        n78 = call-dynamic "Read Camera.lvclass.vi"("error in (no error)"=w216, "Channel in"=w205) -> ("error out"=w212:errorcluster, "Camera.lvclass"=w213:refnum<class "Camera.lvclass">, "Channel out"=w204:refnum<class "Channel.lvclass">)  [unwired: 7 in]
        n79 = call-dynamic "Read SET parameters.vi"("error in (no error)"=w212, "Camera in"=w213) -> ("error out"=w210:errorcluster, "SET parameters"=w207:T8, "Camera out"=w211:refnum<class "Camera.lvclass">)  [unwired: 7 in]
        n80 = Bundle By Name(cluster=w207, "#FRAMES"="Frames") -> (w206:T8)
        n81 = property on="Frames done" class="Slide (strict)"("Scale.Maximum"="Frames") -> ()  [unwired: 2 in, 2 out]
        n82 = call-dynamic "Write SET parameters.vi"("error in (no error)"=w210, "SET parameters"=w206, "Camera in"=w211) -> ("error out"=w208:errorcluster, "Camera out"=w209:refnum<class "Camera.lvclass">)  [unwired: 7 in]
        n83 = call-dynamic "Write Camera.lvclass.vi"("error in (no error)"=w208, "Camera.lvclass"=w209, "Channel in"=w204) -> ("error out"=w215:errorcluster, "Channel out"=w214:refnum<class "Channel.lvclass">)  [unwired: 7 in]
        n84 = call "Write Channel lvclass.vi"("error in (no error)"=w215, "Channel.lvclass"=w214, "SPARC4_GUI in"=w219) -> ("error out"=w202:errorcluster, "SPARC4_GUI out"=w203:refnum<class "S4GEI.lvclass">)  [unwired: 7 in]
        n85 = call "write channel state.vi"("error in (no error)"=w202, "State"="SET_FRAMES", "S4GEI in"=w203) -> ("error out"=w199:errorcluster, "S4GEI out"=w200:refnum<class "S4GEI.lvclass">)  [unwired: 7 in]
      }
      event "Cycles": Value Change {
        n86 = event-data() -> ()  [unwired: 1 in, 6 out]
        n87 = call "Read Channel lvclass.vi"("error in (no error)"=w239, "SPARC4_GUI in"=w240) -> ("error out"=w238:errorcluster, "Channel.lvclass"=w227:refnum<class "Channel.lvclass">, "SPARC4_GUI out"=w241:refnum<class "S4GEI.lvclass">)  [unwired: 7 in]
        n88 = call-dynamic "Read Camera.lvclass.vi"("error in (no error)"=w238, "Channel in"=w227) -> ("error out"=w234:errorcluster, "Camera.lvclass"=w235:refnum<class "Camera.lvclass">, "Channel out"=w226:refnum<class "Channel.lvclass">)  [unwired: 7 in]
        n89 = call-dynamic "Read SET parameters.vi"("error in (no error)"=w234, "Camera in"=w235) -> ("error out"=w232:errorcluster, "SET parameters"=w229:T8, "Camera out"=w233:refnum<class "Camera.lvclass">)  [unwired: 7 in]
        n90 = Bundle By Name(cluster=w229, "#CYCLES"="Cycles") -> (w228:T8)
        n91 = property on="Cycles done" class="Slide (strict)"("Scale.Maximum"="Cycles") -> ()  [unwired: 2 in, 2 out]
        n92 = call-dynamic "Write SET parameters.vi"("error in (no error)"=w232, "SET parameters"=w228, "Camera in"=w233) -> ("error out"=w230:errorcluster, "Camera out"=w231:refnum<class "Camera.lvclass">)  [unwired: 7 in]
        n93 = call-dynamic "Write Camera.lvclass.vi"("error in (no error)"=w230, "Camera.lvclass"=w231, "Channel in"=w226) -> ("error out"=w237:errorcluster, "Channel out"=w236:refnum<class "Channel.lvclass">)  [unwired: 7 in]
        n94 = call "Write Channel lvclass.vi"("error in (no error)"=w237, "Channel.lvclass"=w236, "SPARC4_GUI in"=w241) -> ("error out"=w224:errorcluster, "SPARC4_GUI out"=w225:refnum<class "S4GEI.lvclass">)  [unwired: 7 in]
        n95 = call "write channel state.vi"("error in (no error)"=w224, "State"="SET_CYCLES", "S4GEI in"=w225) -> ("error out"=w221:errorcluster, "S4GEI out"=w222:refnum<class "S4GEI.lvclass">)  [unwired: 7 in]
      }
      event "Suffix": Value Change {
        n96 = event-data() -> ()  [unwired: 1 in, 6 out]
        n97 = call "Read Channel lvclass.vi"("error in (no error)"=w261, "SPARC4_GUI in"=w262) -> ("error out"=w260:errorcluster, "Channel.lvclass"=w249:refnum<class "Channel.lvclass">, "SPARC4_GUI out"=w263:refnum<class "S4GEI.lvclass">)  [unwired: 7 in]
        n98 = call-dynamic "Read Camera.lvclass.vi"("error in (no error)"=w260, "Channel in"=w249) -> ("error out"=w256:errorcluster, "Camera.lvclass"=w257:refnum<class "Camera.lvclass">, "Channel out"=w248:refnum<class "Channel.lvclass">)  [unwired: 7 in]
        n99 = call-dynamic "Read SET parameters.vi"("error in (no error)"=w256, "Camera in"=w257) -> ("error out"=w254:errorcluster, "SET parameters"=w251:T8, "Camera out"=w255:refnum<class "Camera.lvclass">)  [unwired: 7 in]
        n100 = Bundle By Name(cluster=w251, "suffix"="Suffix") -> (w250:T8)
        n101 = call-dynamic "Write SET parameters.vi"("error in (no error)"=w254, "SET parameters"=w250, "Camera in"=w255) -> ("error out"=w252:errorcluster, "Camera out"=w253:refnum<class "Camera.lvclass">)  [unwired: 7 in]
        n102 = call-dynamic "Write Camera.lvclass.vi"("error in (no error)"=w252, "Camera.lvclass"=w253, "Channel in"=w248) -> ("error out"=w259:errorcluster, "Channel out"=w258:refnum<class "Channel.lvclass">)  [unwired: 7 in]
        n103 = call "Write Channel lvclass.vi"("error in (no error)"=w259, "Channel.lvclass"=w258, "SPARC4_GUI in"=w263) -> ("error out"=w246:errorcluster, "SPARC4_GUI out"=w247:refnum<class "S4GEI.lvclass">)  [unwired: 7 in]
        n104 = call "write channel state.vi"("error in (no error)"=w246, "State"="SET_SUFFIX", "S4GEI in"=w247) -> ("error out"=w243:errorcluster, "S4GEI out"=w244:refnum<class "S4GEI.lvclass">)  [unwired: 7 in]
      }
      event "Stop Acquisition": Value Change {
        n105 = event-data() -> ()  [unwired: 1 in, 1 out]
        n106 = flat-sequence {
          tunnel: w264 -> [_]
          frame #0 {
            n107 = local write "Stop Acquisition"(FALSE ("Stop Acquisition")) -> ()
          }
        }
        n108 = call "write channel state.vi"("error in (no error)"=w264, "State"="STOP_ACQUISITION", "S4GEI in"=w268) -> ("error out"=w266:errorcluster, "S4GEI out"=w267:refnum<class "S4GEI.lvclass">)  [unwired: 7 in]
      }
      event "Abort Acquisition": Value Change {
        n109 = event-data() -> ()  [unwired: 1 in, 1 out]
        n110 = call "write channel state.vi"("error in (no error)"=w273, "State"="ABORT_ACQUISITION", "S4GEI in"=w274) -> ("error out"=w270:errorcluster, "S4GEI out"=w272:refnum<class "S4GEI.lvclass">)  [unwired: 7 in]
        n111 = flat-sequence {
          tunnel: w270 -> [_]
          frame #0 {
            n112 = local write "Abort Acquisition"(FALSE ("Abort Acquisition")) -> ()
          }
        }
      }
      event "Pause acquisition": Value Change {
        n113 = event-data() -> ()  [unwired: 1 in, 1 out]
        n114 = Select(t="PAUSE_ACQUISITION", s="Pause acquisition", f="RESUME_ACQUISITION") -> (s? t:f=w278:string)
        n115 = call "write channel state.vi"("error in (no error)"=w282, "State"=w278, "S4GEI in"=w283) -> ("error out"=w280:errorcluster, "S4GEI out"=w281:refnum<class "S4GEI.lvclass">)  [unwired: 7 in]
      }
      event "comment": Value Change {
        n116 = event-data() -> ()  [unwired: 1 in, 6 out]
        n117 = call-dynamic "Read GEI status.vi"("error in (no error)"=w289, "S4GEI in"=w291) -> ("error out"=w287:errorcluster, "GEI status"=w288:T9, "S4GEI out"=w286:refnum<class "S4GEI.lvclass">)  [unwired: 7 in]
        n118 = Bundle By Name(cluster=w288, "COMMENT"="comment") -> (w285:T9)
        n119 = call-dynamic "Write GEI status.vi"("error in (no error)"=w287, "GEI status"=w285, "S4GEI in"=w286) -> ("error out"=w290:errorcluster, "S4GEI out"=w292:refnum<class "S4GEI.lvclass">)  [unwired: 7 in]
      }
      event "Object name": Value Change {
        n120 = event-data() -> ()  [unwired: 1 in, 6 out]
        n121 = call-dynamic "Read GEI status.vi"("error in (no error)"=w298, "S4GEI in"=w300) -> ("error out"=w296:errorcluster, "GEI status"=w297:T9, "S4GEI out"=w295:refnum<class "S4GEI.lvclass">)  [unwired: 7 in]
        n122 = Bundle By Name(cluster=w297, "OBJECT"="Object name") -> (w294:T9)
        n123 = call-dynamic "Write GEI status.vi"("error in (no error)"=w296, "GEI status"=w294, "S4GEI in"=w295) -> ("error out"=w299:errorcluster, "S4GEI out"=w301:refnum<class "S4GEI.lvclass">)  [unwired: 7 in]
      }
      event "PROPID": Value Change {
        n124 = event-data() -> ()  [unwired: 1 in, 6 out]
        n125 = call-dynamic "Read GEI status.vi"("error in (no error)"=w307, "S4GEI in"=w309) -> ("error out"=w305:errorcluster, "GEI status"=w306:T9, "S4GEI out"=w304:refnum<class "S4GEI.lvclass">)  [unwired: 7 in]
        n126 = Bundle By Name(cluster=w306, "PROJID"="PROPID") -> (w303:T9)
        n127 = call-dynamic "Write GEI status.vi"("error in (no error)"=w305, "GEI status"=w303, "S4GEI in"=w304) -> ("error out"=w308:errorcluster, "S4GEI out"=w310:refnum<class "S4GEI.lvclass">)  [unwired: 7 in]
      }
      event "Observer": Value Change {
        n128 = event-data() -> ()  [unwired: 1 in, 6 out]
        n129 = call-dynamic "Read GEI status.vi"("error in (no error)"=w316, "S4GEI in"=w318) -> ("error out"=w314:errorcluster, "GEI status"=w315:T9, "S4GEI out"=w313:refnum<class "S4GEI.lvclass">)  [unwired: 7 in]
        n130 = Bundle By Name(cluster=w315, "OBSERVER"="Observer") -> (w312:T9)
        n131 = call-dynamic "Write GEI status.vi"("error in (no error)"=w314, "GEI status"=w312, "S4GEI in"=w313) -> ("error out"=w317:errorcluster, "S4GEI out"=w319:refnum<class "S4GEI.lvclass">)  [unwired: 7 in]
      }
      event "Sub Image": Value Change {
        n132 = event-data() -> ()  [unwired: 1 in, 1 out]
        n133 = Divide(x=2048, y=2) -> (x/y=w320:dbl)
        n134 = case shown="\"512 x 512\"" "Sub Image" {
          tunnel: [256 512 1024 512] -> w326
          frame "512 x 512" {
          }
          frame "1024 x 1024" {
          }
          frame "2048 x 2048", Default {
          }
          frame "Custom" {
          }
        }
        n135 = case shown="\"Custom\"" "Sub Image" {
          tunnel: [T3."Disabled and Grayed Out" ("Disabled") T3."Enabled" ("Disabled")] -> w329
          frame "1024 x 1024", Default {
          }
          frame "Custom" {
          }
        }
        n136 = Add(x=w320, y=w326) -> (x+y=w322:dbl)
        n137 = Subtract(x=w320, y=w326) -> (x-y=w327:dbl)
        n138 = Subtract(x=w320, y=w326) -> (x-y=w328:dbl)
        n139 = Add(x=w320, y=w326) -> (x+y=w331:dbl)
        n140 = Increment(x=w327) -> (x+1=w330:dbl)
        n141 = Increment(x=w328) -> (x+1=w323:dbl)
        n142 = local write "Initial Cloumn"(w330) -> ()
        n143 = local write "Final Column"(w331) -> ()
        n144 = local write "Initial Line"(w323) -> ()
        n145 = local write "Final Line"(w322) -> ()
        n146 = property on="Initial Line" class="DigNum (strict)"("DisabledEnum"=w329) -> ()  [unwired: 2 in, 2 out]
        n147 = property on="Initial Cloumn" class="DigNum (strict)"("DisabledEnum"=w329) -> ()  [unwired: 2 in, 2 out]
        n148 = property on="Final Line" class="DigNum (strict)"("DisabledEnum"=w329) -> ()  [unwired: 2 in, 2 out]
        n149 = property on="Final Column" class="DigNum (strict)"("DisabledEnum"=w329) -> ()  [unwired: 2 in, 2 out]
        n150 = flat-sequence {
          tunnel: w334 -> [w352]
          tunnel: w335 -> [w353]
          tunnel: [w353] -> w333
          tunnel: [w352] -> w332
          frame #0 {
            w346 = cluster{dbl, dbl} {0.0, 0.0}
            n151 = local read "Initial Cloumn"() -> (w345:u16)
            n152 = local read "Final Column"() -> (w343:u16)
            n153 = local read "Final Line"() -> (w344:u16)
            n154 = local read "Final Line"() -> (w342:u16)
            n155 = Bundle(cluster=w346, w345, w344) -> (w351:cluster{dbl, dbl})
            n156 = Bundle(cluster=w346, w345, w342) -> (w350:cluster{dbl, dbl})
            n157 = Bundle(cluster=w346, w343, w342) -> (w349:cluster{dbl, dbl})
            n158 = Bundle(cluster=w346, w343, w344) -> (w348:cluster{dbl, dbl})
            n159 = Bundle(cluster=w346, w345, w344) -> (w347:cluster{dbl, dbl})
            n160 = Build Array(w351, w350, w349, w348, w347) -> ()  [unwired: 1 out]
          }
        }
      }
      event "Acquisition Mode": Value Change {
        n161 = event-data() -> ("NewVal"=w355:u16)  [unwired: 1 in]
        n162 = case shown="1, Default" w355 {
          tunnel: [T3."Enabled" ("Disabled") T3."Disabled and Grayed Out" ("Disabled")] -> w354
          frame 3 {
          }
          frame 1, Default {
          }
        }
        n163 = property on="Frames" class="DigNum (strict)"("DisabledEnum"=w354) -> ()  [unwired: 2 in, 2 out]
      }
    }
    n164 = Unbundle By Name(w13) -> ("status"=w18:bool)
    n165 = Or(x=w18, y="Stop Application") -> (x .or. y?=w19:bool)
  }
  n166 = Unbundle By Name(w9) -> ("source"=→"Error Message":string)
  n167 = call <vilib>:"Clear Errors.vi"("error in (no error)"=w9) -> ("error out"=w8:errorcluster)  [unwired: 5 in, 1 out]
  n168 = call "End.vi"("error in (no error)"=w8, "SPARC4_GUI in"=w11) -> ("SPARC4_GUI out"=w12:refnum<class "S4GEI.lvclass">)  [unwired: 8 in, 1 out]
  n169 = flat-sequence {
    tunnel: w12 -> [_]
    frame #0 {
      w362 = 1
      w364 = ""
      w365 = FALSE ("analyser status")
      (unwired) 0.0 ("Scale.Range:Minimum")
      (unwired) 1.0 ("Scale.Range:Maximum")
      (unwired) 1.0 ("Scale.Range:Maximum")
      (unwired) T3."Disabled and Grayed Out" ("Disabled")
      w369 = u16 0 items=["Internal", "External", "N/A", "N/A", "N/A", "N/A", "External Start", "External Exposure (Bulb)", "N/A", "External FVB EM", "Software", "N/A", "External Charge Shifting"] ("Trigger Mode")
      w370 = u16 4 items=["Full Vertical Binning", "Multi-Track", "Random-Track", "Single-Track", "Image"] ("Read Mode")
      w371 = u16 3 items=["Reserved", "Single Scan", "Accumulate", "Kinetic", "Fast Kinetic", "Run till abort", "Reserved", "Reserved", "Reserved", "Time Delayed Integration"] ("Acquisition Mode")
      w376 = u16 0 items=["TTL Low", "TTL High"] ("Shutter TTL")
      w377 = u8 0 items=["  1 MHz", "0.1 MHz"] ("Readout Rate")
      w379 = u8 2 items=["Fully Auto", "OPEN", "CLOSED"] ("Shutter Mode")
      w363 = "" ("Command:")
      w381 = u16 2048 ("Final Line")
      w380 = u16 1 ("Initial Cloumn")
      w383 = u8 0 items=["Gain 1", "Gain 2"] ("Pre-amp gain")
      n170 = local write "Frames"(w362) -> ()
      n171 = local write "Cycles"(w362) -> ()
      n172 = property on="Cycles done" class="Slide (strict)"("Scale.Maximum"=1.0 ("Scale.Range:Maximum")) -> ()  [unwired: 2 in, 2 out]
      n173 = property on="Frames done" class="Slide (strict)"("Scale.Maximum"=1.0 ("Scale.Range:Maximum")) -> ()  [unwired: 2 in, 2 out]
      n174 = property on="Temperature" class="DigNum (strict)"("NumText.BGColor"=u32 12369084) -> ()  [unwired: 2 in, 2 out]
      n175 = local write "PROPID"(w363) -> ()
      n176 = local write "Observer"(w363) -> ()
      n177 = local write "Object name"(w364) -> ()
      n178 = local write "comment"(w364) -> ()
      n179 = property on="ACS mode" class="Bool (strict)"("Colors [4]"=cluster{u32, u32}[] [{1985280, 1985280}, {1985280, 1985280}, {6618880, 6618880}]) -> ()  [unwired: 2 in, 2 out]
      n180 = local write "Start exposure"(w365) -> ()
      n181 = local write "Stop Acquisition"(w365) -> ()
      n182 = local write "Abort Acquisition"(w365) -> ()
      n183 = local write "Pause acquisition"(w365) -> ()
      n184 = local write "Shutter TTL"(w376) -> ()
      n185 = local write "Shutter Time"(u16 50 ("Shutter Time")) -> ()
      n186 = local write "AD Channel"(u16 0 ("AD Channel")) -> ()
      n187 = local write "Acquisition Mode"(w371) -> ()
      n188 = local write "Read Mode"(w370) -> ()
      n189 = local write "Trigger Mode"(w369) -> ()
      n190 = local write "Shutter Mode"(w379) -> ()
      n191 = local write "VShift Speed"(u16 0 ("Vertical Shift Speed")) -> ()
      n192 = local write "Clock Amplitude"(u16 0 ("Vertical Clock Voltagem")) -> ()
      n193 = local write "Readout Rate"(w377) -> ()
      n194 = local write "Pre-amp gain"(w383) -> ()
      n195 = local write "Sub Image"(T1."2048 x 2048" ("Sub Image")) -> ()
      n196 = local write "Initial Line"(u16 1 ("Initial Line")) -> ()
      n197 = local write "Final Line"(w381) -> ()
      n198 = local write "Final Column"(w381) -> ()
      n199 = local write "Initial Cloumn"(w380) -> ()
      n200 = local write "Binning"(w380) -> ()
      n201 = property on="Frames" class="DigNum (strict)"("DisabledEnum"=T3."Enabled" ("Disabled")) -> ()  [unwired: 2 in, 2 out]
    }
  }
